vi "Get Device Adresses (SubVI).vi"(8 "error in (no error)":errorcluster, 10 "DeviceKey In":string, 11 "CmdLib In":refnum<k24>) -> (0 "error out":errorcluster, 1 "Device Addresses":i32[](array[numeric]), 2 "DeviceKey Out":string, 3 "CmdLib Out":refnum<k24>)   [LabVIEW 2017]
uses:
  dll/CmdLib.dll
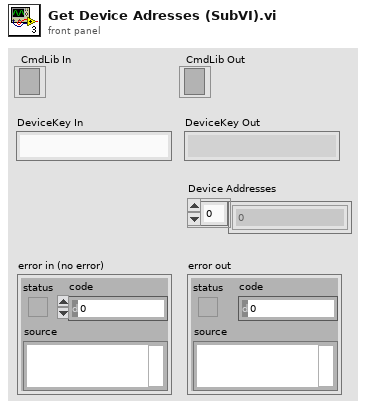
[diagram p1: front panel]
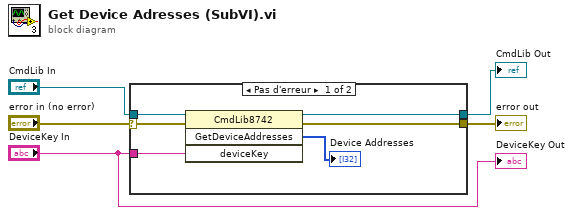
[diagram p0: block diagram]
diagram:
  n1 = case shown="Pas d'erreur" "error in (no error)" {
    selector: "error in (no error)" -> [w8 w13]
    tunnel: "CmdLib In" -> [w11 w12]
    tunnel: [w10 w12] -> w4
    tunnel: "DeviceKey In" -> [w9 _]
    tunnel: [w6 w13] -> w1
    frame No Error {
      n2 = invoke class="CmdLib8742" method="GetDeviceAddresses"(reference=w11, error in=w8, "deviceKey"=w9) -> (reference out=w10:refnum<k24>, error out=w6:errorcluster, "GetDeviceAddresses"=→"Device Addresses":i32[])  [unwired: 1 in, 1 out]
    }
    frame Error {
    }
  }
  "CmdLib Out" <- w4
  "error out" <- w1
  "DeviceKey Out" <- "DeviceKey In"
